vi "Create Table Query.vi"(8 "error in (no error)":errorcluster, 9 "Column Definition Strings":string[](array[string]), 10 "Table Name":string, 11 "DatabaseBaseClass in":refnum<class "DatabaseBaseClass.lvclass">) -> (0 "error out":errorcluster, 1 "Create Table Query":string, 3 "DatabaseBaseClass out":refnum<class "DatabaseBaseClass.lvclass">)   [LabVIEW 2018, in "Database.lvlib" / "DatabaseBaseClass.lvclass"]
uses:
  DatabaseBaseClass.lvclass
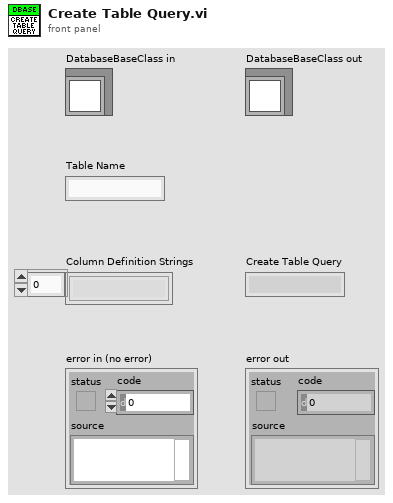
[diagram p1: front panel]
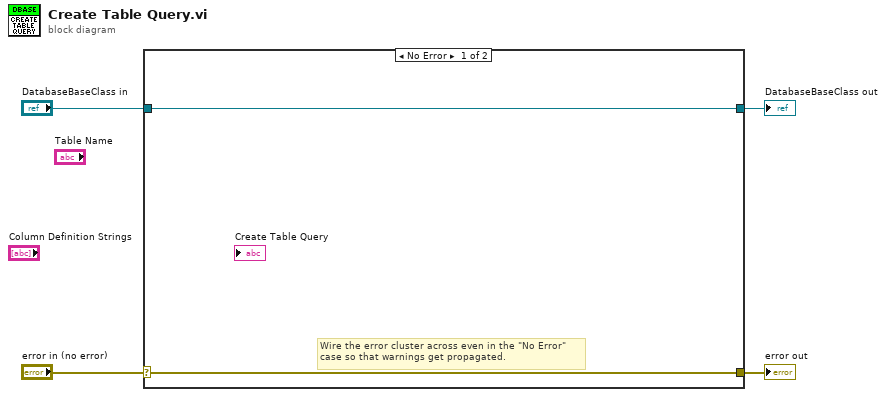
[diagram p0: block diagram]
diagram:
  n1 = case shown="No Error" "error in (no error)" {
    selector: "error in (no error)" -> [w5 w8]
    tunnel: [w5 w8] -> w3
    tunnel: [w6 w7] -> w1
    tunnel: "DatabaseBaseClass in" -> [w6 w7]
    frame No Error {
      # "Wire the error cluster across even in the \"No Error\"\ncase so that warnings get propagated."
    }
    frame Error {
    }
  }
  "error out" <- w3
  "DatabaseBaseClass out" <- w1
